vi "TeleopAuto.vi"(11 "Counts":dbl) -> ()   [LabVIEW 2018]
uses:
  <vilib>/Rock Robotics/WPI/Solenoid/WPI_SolenoidValue.ctl
  <vilib>/Rock Robotics/WPI/ThirdParty/Phoenix-LabVIEW/Motor Controller/Controls/CTRE_Phoenix_MotorControl_ControlMode.ctl
  <vilib>/Rock Robotics/WPI/Utilities/WPI_GetSetVariantRefNum.vi
  <vilib>/Rock Robotics/Network Tables/NT Write Boolean Array.vi
  <vilib>/Rock Robotics/Network Tables/NT Write Numeric Array.vi
  <vilib>/Rock Robotics/WPI/Solenoid/WPI_SolenoidSetEnum.vi
  <vilib>/Rock Robotics/Network Tables/NT Write Boolean.vi
  <vilib>/Rock Robotics/WPI/ThirdParty/Phoenix-LabVIEW/Motor Controller/Get/CTRE_Phoenix_MotorController_GetQuadratureData.vi
  <vilib>/Rock Robotics/Network Tables/NT Write Number.vi
  <vilib>/Rock Robotics/Network Tables/NT Read Number.vi
panel:
  out "Angle Ref":dbl
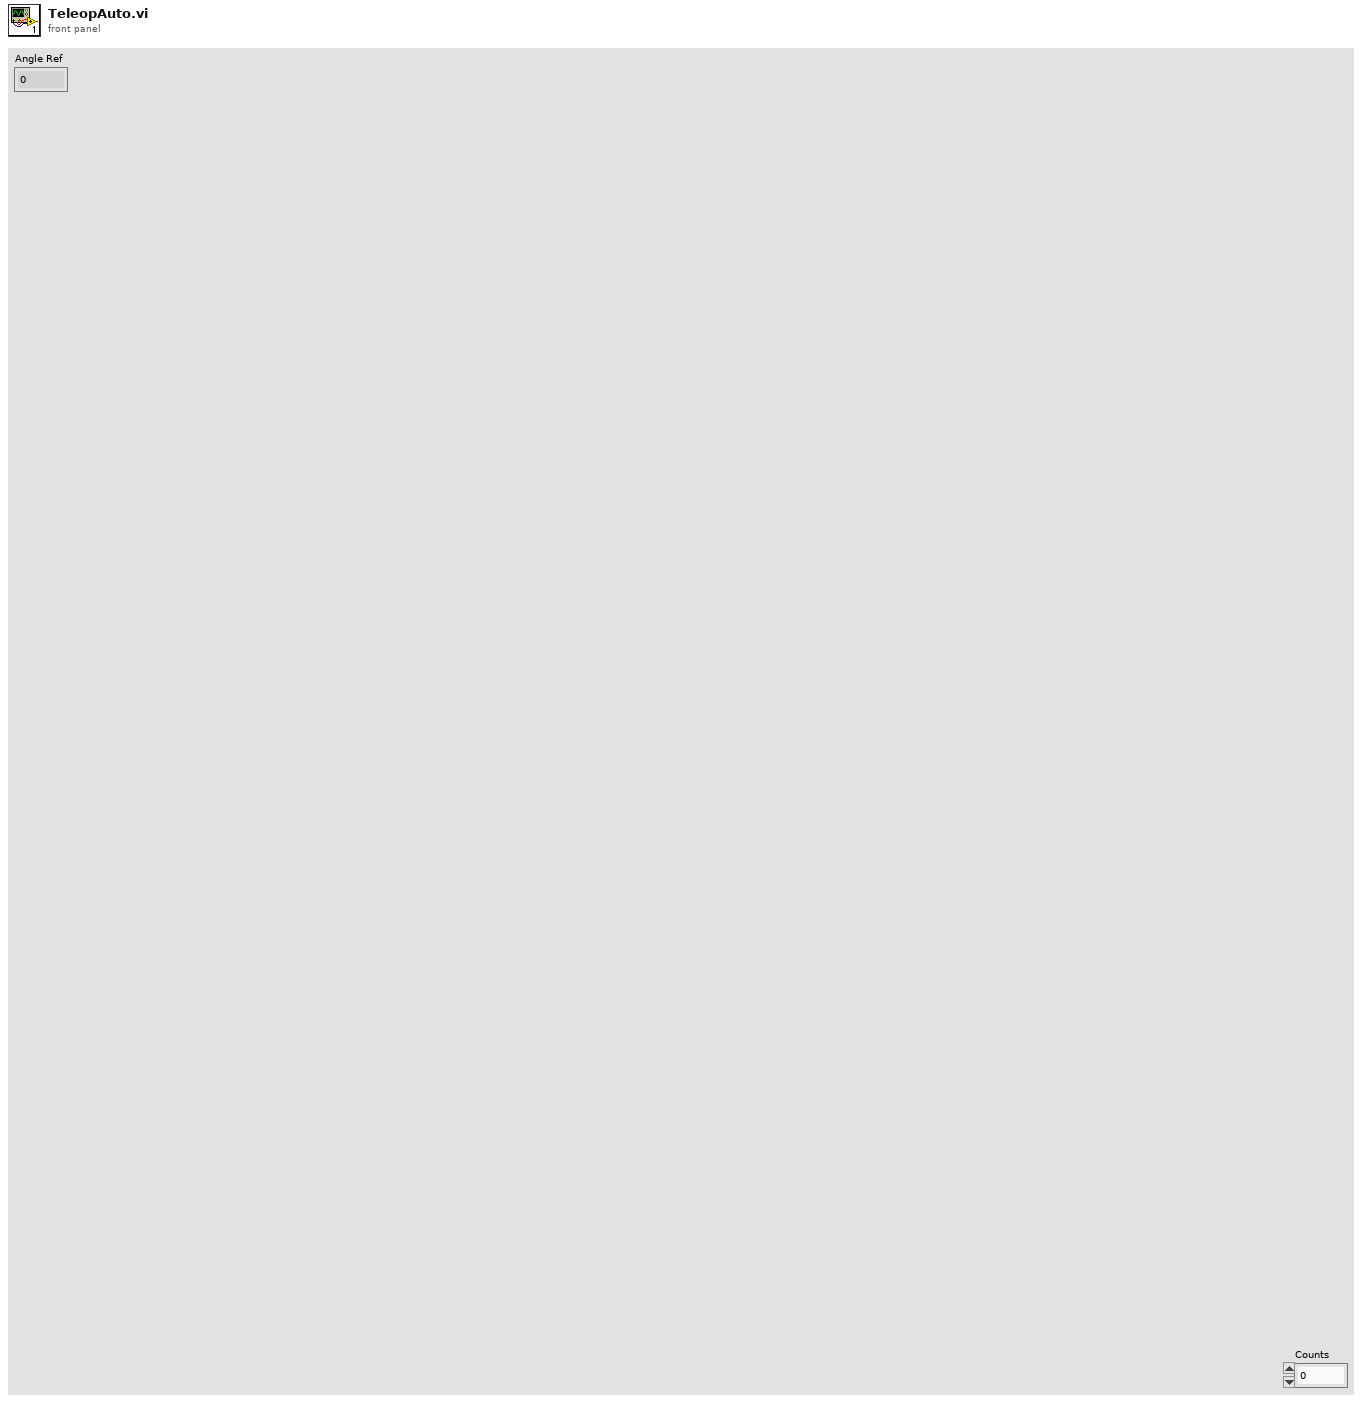
[diagram p1: front panel]
types:
  T1 = typedef "CTRE_Phoenix_MotorControl_ControlMode.ctl" = u16
  T2 = typedef "WPI_SolenoidValue.ctl" = enum16{"Off", "On", "Forward", "Reverse"}
  T3 = typedef "WPI_JoystickDevRef.ctl" = cluster{"Device":T4}
  T4 = typedef "WPI_JoystickDeviceEnum.ctl" = enum16{"USB 0", "USB 1", "USB 2", "USB 3", "USB 4", "USB 5"}
  T5 = cluster{"Buttons[0]":bool, "Buttons[1]":bool, "Buttons[2]":bool, "Buttons[3]":bool, "Buttons[4]":bool, "Buttons[5]":bool, "Buttons[6]":bool, "Buttons[7]":bool, "Buttons[8]":bool, "Buttons[9]":bool, "Buttons[10]":bool, "Buttons[11]":bool, "Buttons[12]":bool, "Buttons[13]":bool}
  T6 = cluster{"Axes[0]":dbl, "Axes[1]":dbl, "Axes[2]":dbl, "Axes[3]":dbl, "Axes[4]":dbl, "Axes[5]":dbl, "Axes[6]":dbl, "Axes[7]":dbl, "Axes[8]":dbl}
  T7 = typedef "WPI_SolenoidDevRef.ctl" = cluster{"DevStatus":errorcluster, "Pneumatics Control Module":u8, "Forward Solenoid Channel":T8, "Reverse Solenoid Channel":T8}
  T8 = typedef "WPI_SolenoidChannel.ctl" = enum8{"Solenoid 0", "Solenoid 1", "Solenoid 2", "Solenoid 3", "Solenoid 4", "Solenoid 5", "Solenoid 6", "Solenoid 7", "Invalid"}
  T9 = cluster{"Yaw":dbl, "Roll":dbl, "Pitch":dbl, "Heading":dbl, "Fused Heading":dbl}
  T10 = typedef "WPI_MotorControlDeviceRef.ctl" = cluster{"DeviceStatus":errorcluster, "Type":T11, "PWM":cluster{"PWM Channel":T12, "DeadBand":T13}, "CAN":cluster{"Device Number":u8, "SetOutput VI Ref":variant, "GetOutput VI Ref":variant, "Enable VI Ref":variant, "Disable VI Ref":variant, "Data":variant}, "Invert":bool, "DIO PWM":cluster{"PWM \"Enable\" Channel":T12, "DIOChannel":T14, "PWM Rate":dbl}}
  T11 = typedef "WPI_MotorControlType.ctl" = enum16{"PWM", "CAN", "DIO PWM"}
  T12 = typedef "FPGA_DIOPWMChannel.ctl" = enum8{"PWM 0", "PWM 1", "PWM 2", "PWM 3", "PWM 4", "PWM 5", "PWM 6", "PWM 7", "PWM 8", "PWM 9", "PWM MXP 0", "PWM MXP 1", "PWM MXP 2", "PWM MXP 3", "PWM MXP 4", "PWM MXP 5", "PWM MXP 6", "PWM MXP 7", "PWM MXP 8", "PWM MXP 9", "Invalid"}
  T13 = typedef "WPI_PWMDeadband.ctl" = cluster{"Name":string, "maxPositivePwm":i32, "minPositivePwm":i32, "centerPwm":i32, "maxNegativePwm":i32, "minNegativePwm":i32, "angularRange":u16}
  T14 = typedef "FPGA_DIOChannel.ctl" = enum8{"DIO 0", "DIO 1", "DIO 2", "DIO 3", "DIO 4", "DIO 5", "DIO 6", "DIO 7", "DIO 8", "DIO 9", "DIO MXP 0", "DIO MXP 1", "DIO MXP 2", "DIO MXP 3", "DIO MXP 4", "DIO MXP 5", "DIO MXP 6", "DIO MXP 7", "DIO MXP 8", "DIO MXP 9", "DIO MXP 10", "DIO MXP 11", "DIO MXP 12", "DIO MXP 13", "DIO MXP 14", "DIO MXP 15", "SPI Port CS1", "SPI Port CS2", "SPI Port CS3", "SPI Port MISO", "SPI Port MOSI", "Invalid"}
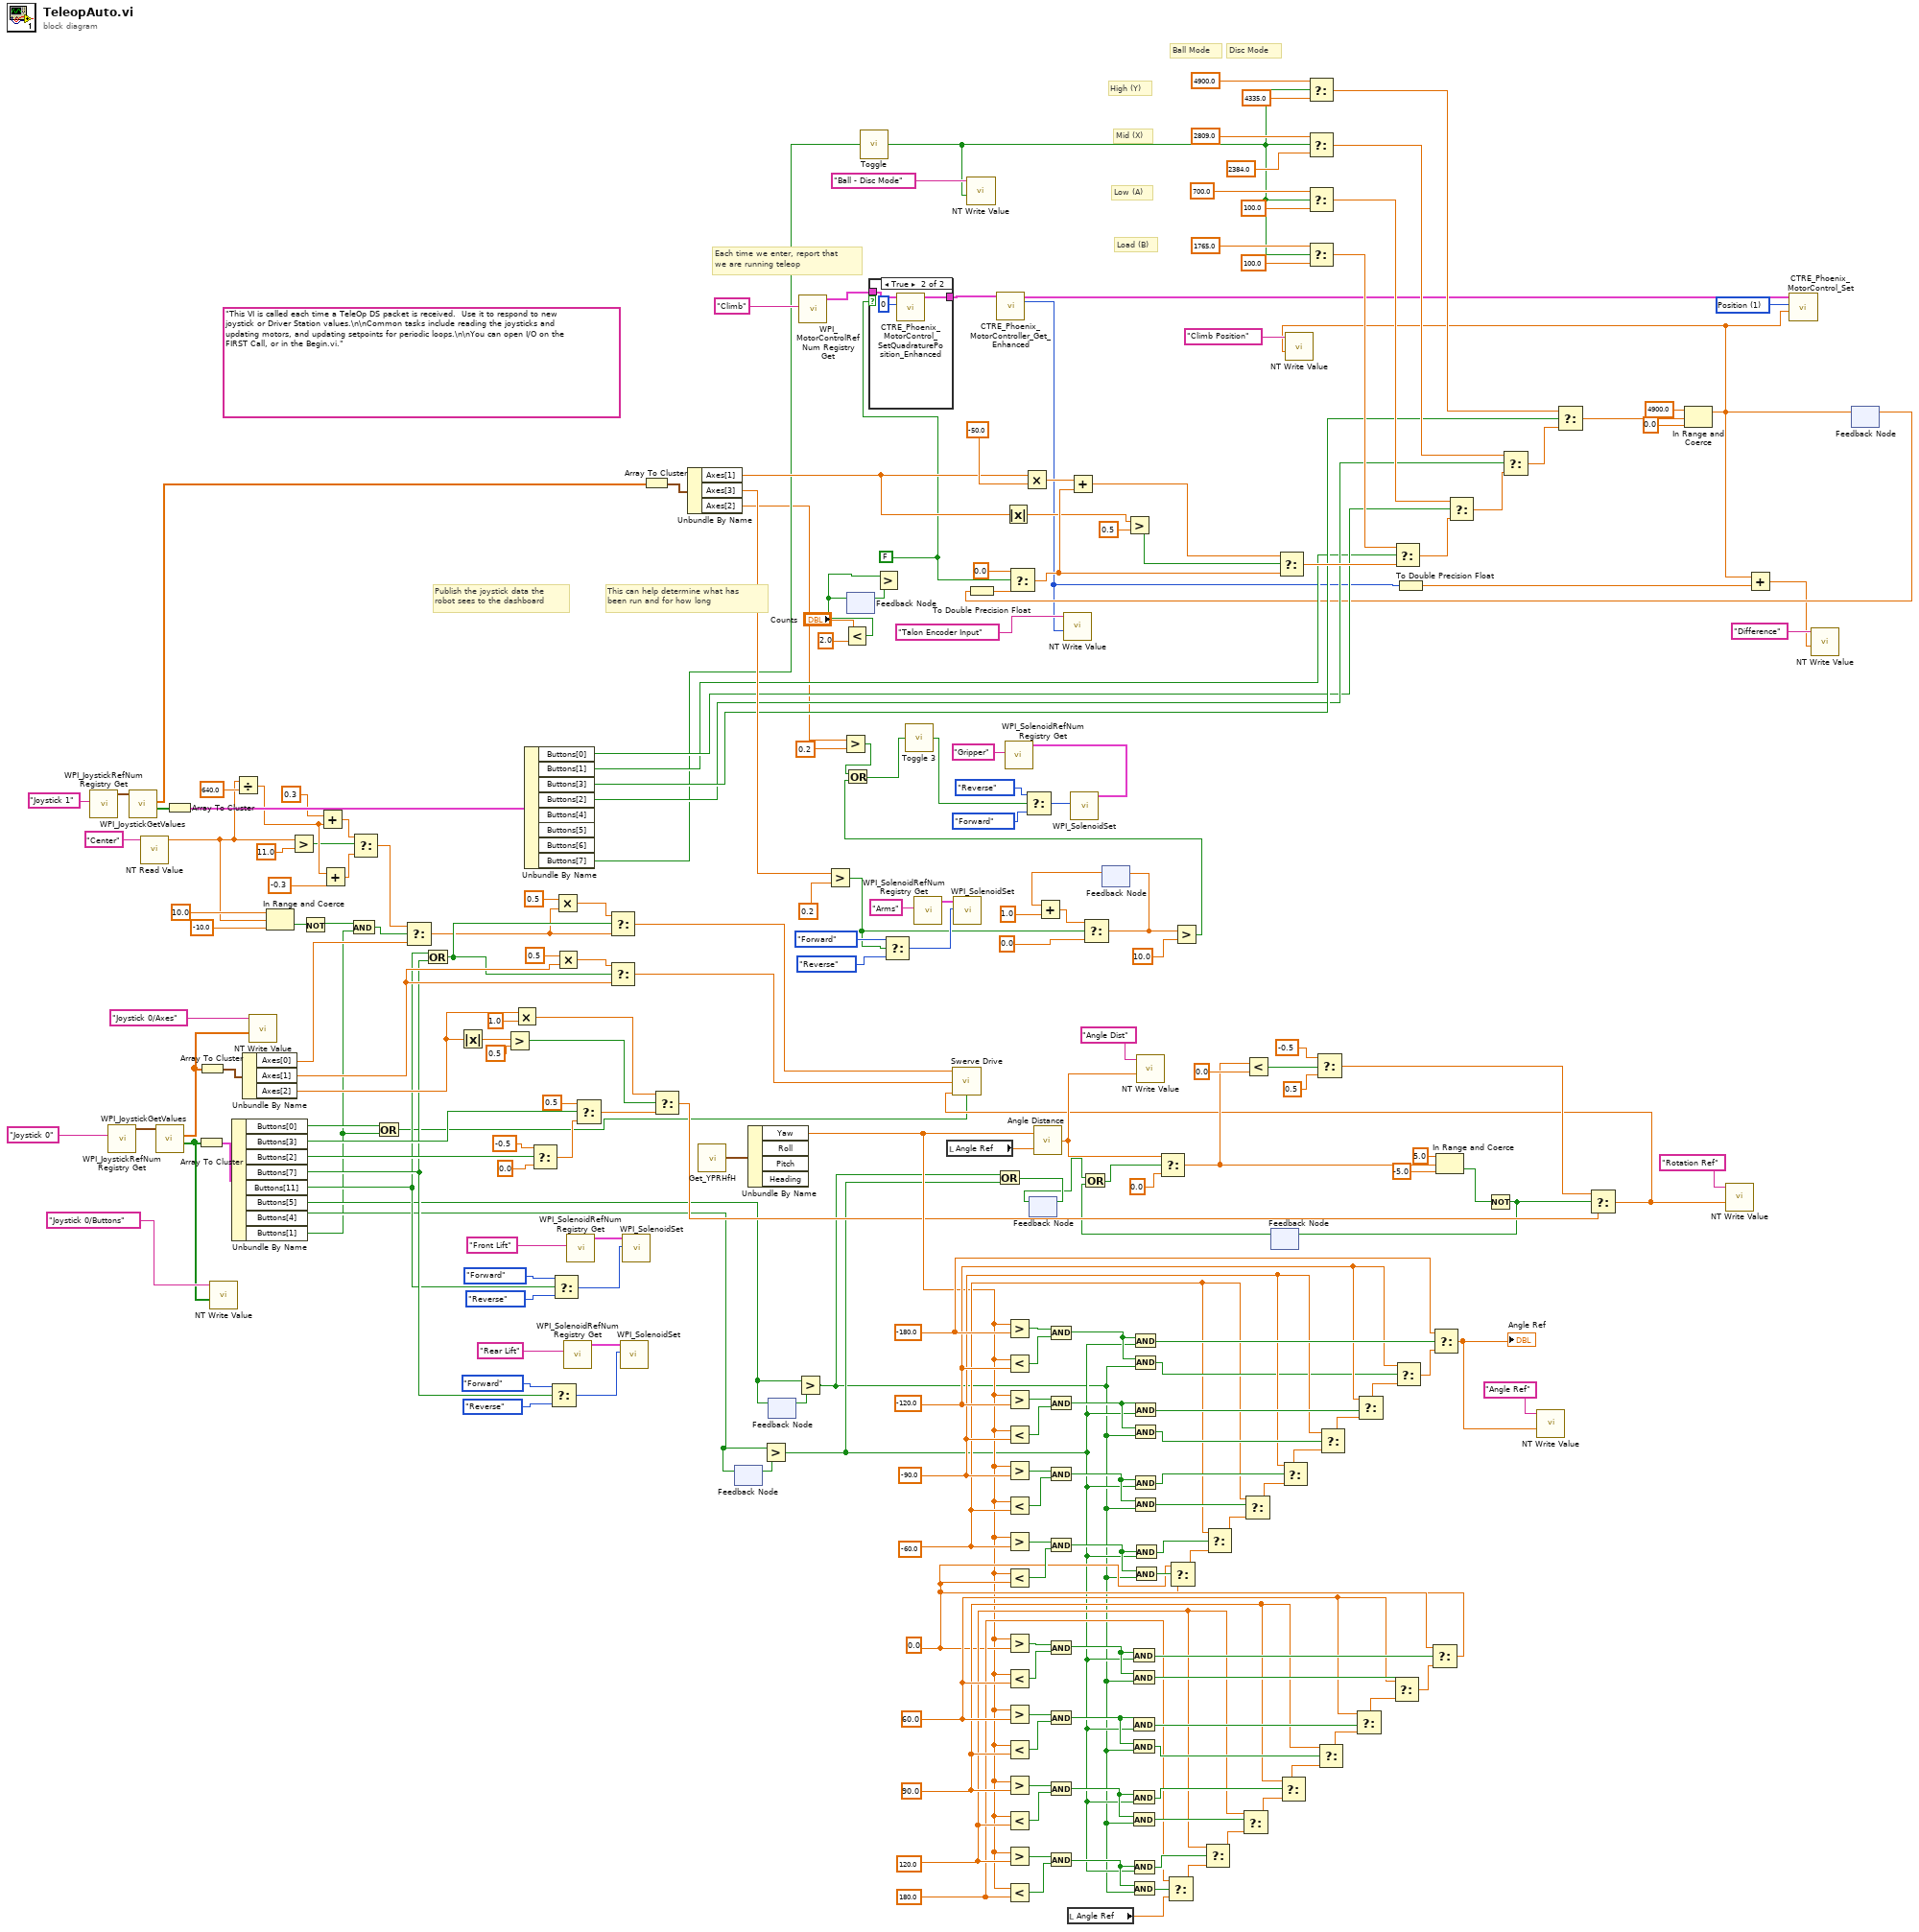
[diagram p0: block diagram]
diagram:
  w35 = FALSE
  w65 = -180.0
  w64 = -120.0
  w63 = -90.0
  w59 = -60.0
  w92 = 180.0
  w93 = 120.0
  w94 = 90.0
  w95 = 60.0
  w62 = 0.0
  w209 = T1 1 items=["PercentOutput"=0, "Position"=1, "Velocity"=2, "Current"=3, "Follower"=5, "MotionProfile"=6, "MotionMagic"=7, "MotionProfileArc"=10, "Disabled"=15] ("Control Mode")
  (unwired) "This VI is called each time a TeleOp DS packet is received.  Use it to respond to new joystick or Driver Station values.\n\nCommon tasks include reading the joysticks and updating motors, and updating setpoints for periodic loops.\n\nYou can open I/O on the FIRST Call, or in the Begin.vi."
  # "High (Y)"
  # "Mid (X)"
  # "Low (A)"
  # "Load (B)"
  # "Disc Mode"
  # "Ball Mode"
  # "Publish the joystick data the\nrobot sees to the dashboard"
  # "Each time we enter, report that\nwe are running teleop"
  # "This can help determine what has\nbeen run and for how long"
  n1 = call <vilib>:"WPI_JoystickRefNum Registry Get.vi"("refnum name"="Joystick 1") -> ("JoystickDevRef"=w216:T3)  [unwired: 1 in, 9 out]
  n2 = call <vilib>:"WPI_JoystickRefNum Registry Get.vi"("refnum name"="Joystick 0") -> ("JoystickDevRef"=w242:T3)  [unwired: 1 in, 9 out]
  n3 = call <vilib>:"WPI_JoystickGetValues.vi"("JoystickDevRef"=w216) -> ("Buttons"=w214:bool[], "Axes"=w210:dbl[])  [unwired: 6 in, 3 out]
  n4 = call-poly <vilib>:"NT Read Value.vi"("Name"="Center" ("refnum name")) -> ("Numeric"=w6:dbl)  [unwired: 9 in, 1 out]
  n5 = call <vilib>:"WPI_JoystickGetValues.vi"("JoystickDevRef"=w242) -> ("Buttons"=w237:bool[], "Axes"=w239:dbl[])  [unwired: 6 in, 3 out]
  n6 = Array To Cluster(array=w214) -> (cluster=w213:T5)
  n7 = Array To Cluster(array=w237) -> (cluster=w236:T5)
  n8 = Array To Cluster(array=w239) -> (cluster=w238:T6)
  n9 = call-poly <vilib>:"NT Write Value.vi"("Boolean Array"=w237, "Name"="Joystick 0/Buttons") -> ()  [unwired: 9 in, 1 out]
  n10 = Unbundle By Name(w236) -> ("Buttons[0]"=w20:bool, "Buttons[3]"=w134:bool, "Buttons[2]"=w135:bool, "Buttons[7]"=w52:bool, "Buttons[11]"=w51:bool, "Buttons[5]"=w34:bool, "Buttons[4]"=w32:bool, "Buttons[1]"=w16:bool)
  n11 = Divide(x=w6, y=640.0) -> (x/y=w5:dbl)
  n12 = Unbundle By Name(w238) -> ("Axes[0]"=w24:dbl, "Axes[1]"=w54:dbl, "Axes[2]"=w141:dbl)
  n13 = call-poly <vilib>:"NT Write Value.vi"("Numeric Array"=w239, "Name"="Joystick 0/Axes") -> ()  [unwired: 9 in, 1 out]
  n14 = In Range and Coerce(upper limit=10.0, x=w6, lower limit=-10.0) -> (In Range?=w14:bool)  [unwired: 1 out]
  n15 = Greater?(x=w6, y=11.0) -> (0:w4:bool)
  n16 = Not(x=w14) -> (.not. x?=w15:bool)
  n17 = Add(x=0.3 ("t"), y=w5) -> (x+y=w10:dbl)
  n18 = Add(x=w5, y=-0.3 ("f")) -> (x+y=w11:dbl)
  n19 = And(x=w15, y=w16) -> (x .and. y?=w13:bool)
  n20 = Select(t=w10, s=w4, f=w11) -> (s? t:f=w22:dbl)
  n21 = Or(x=w20, y=w16) -> (x .or. y?=w19:bool)
  n22 = Select(t=w22, s=w13, f=w24) -> (s? t:f=w23:dbl)
  n23 = Or(x=w51, y=w52) -> (x .or. y?=w50:bool)
  n24 = Absolute Value(x=w141) -> (abs(x)=w144:dbl)
  n25 = Greater?(x=w144, y=0.5) -> (0:w133:bool)
  n26 = Multiply(x=w141, y=1.0) -> (x*y=w142:dbl)
  n27 = Unbundle By Name(w213) -> ("Buttons[0]"=w175:bool, "Buttons[1]"=w174:bool, "Buttons[3]"=w177:bool, "Buttons[2]"=w176:bool, "Buttons[7]"=w172:bool)  [unwired: 3 out]
  n28 = Select(t=-0.5, s=w135, f=0.0) -> (s? t:f=w139:dbl)
  n29 = Select(t=WPI_SolenoidValue."Forward" ("Value"), s=w52, f=WPI_SolenoidValue."Reverse") -> (s? t:f=w219:T2)
  n30 = Select(t=WPI_SolenoidValue."Forward" ("Value"), s=w51, f=WPI_SolenoidValue."Reverse") -> (s? t:f=w218:T2)
  n31 = Multiply(x=0.5, y=w23) -> (x*y=w53:dbl)
  n32 = Multiply(x=0.5, y=w54) -> (x*y=w55:dbl)
  n33 = call <vilib>:"WPI_SolenoidRefNum Registry Get.vi"("refnum name"="Rear Lift") -> ("SolenoidDevRef"=w229:T7)  [unwired: 9 in, 1 out]
  n34 = call <vilib>:"WPI_SolenoidRefNum Registry Get.vi"("refnum name"="Front Lift") -> ("SolenoidDevRef"=w230:T7)  [unwired: 9 in, 1 out]
  n35 = Select(t=0.5, s=w134, f=w139) -> (s? t:f=w132:dbl)
  n36 = Select(t=w53, s=w50, f=w23) -> (s? t:f=w48:dbl)
  n37 = Select(t=w55, s=w50, f=w54) -> (s? t:f=w49:dbl)
  n38 = call-poly <vilib>:"WPI_SolenoidSet.vi"("Value"=w219, "SolenoidDevRef"=w229) -> ()  [unwired: 8 in, 2 out]
  n39 = call-poly <vilib>:"WPI_SolenoidSet.vi"("Value"=w218, "SolenoidDevRef"=w230) -> ()  [unwired: 8 in, 2 out]
  n40 = Array To Cluster(array=w210) -> (cluster=w211:T6)
  n41 = Select(t=w142, s=w133, f=w132) -> (s? t:f=w43:dbl)
  n42 = Unbundle By Name(w211) -> ("Axes[1]"=w197:dbl, "Axes[3]"=w204:dbl, "Axes[2]"=w170:dbl)
  n43 = call <vilib>:"Get_YPRHfH.vi"() -> ("YRPHfH"=w131:T9)  [unwired: 11 in]
  n44 = feedback #1() -> (w45:bool)  [unwired: 1 in]
  n45 = feedback-in #1(w32) -> ()
  n46 = Unbundle By Name(w131) -> ("Yaw"=w58:dbl)  [unwired: 3 out]
  n47 = Greater?(x=w32, y=w45) -> (0:w26:bool)
  n48 = feedback #2() -> (w46:bool)  [unwired: 1 in]
  n49 = feedback-in #2(w34) -> ()
  n50 = Greater?(x=w34, y=w46) -> (0:w25:bool)
  n51 = call <vilib>:"WPI_MotorControlRefNum Registry Get.vi"("refnum name"="Climb") -> ("MotorControlDevRef"=w155:T10)  [unwired: 9 in, 1 out]
  n52 = Greater?(x=w204, y=0.2) -> (0:w167:bool)
  n53 = Greater?(x=w170, y=0.2) -> (0:w160:bool)
  n54 = Less?(x="Counts", y=2.0) -> (x < y?=w2:bool)
  n55 = feedback #3() -> (w153:bool)  [unwired: 1 in]
  n56 = feedback-in #3(w2) -> ()
  n57 = call "Toggle.vi"("Input"=w172) -> ("Output"=w157:bool)
  n58 = case shown="True" w35 {
    tunnel: w155 -> [w244 w247]
    tunnel: [w244 w246] -> w154
    frame False {
    }
    frame True {
      n59 = call <vilib>:"CTRE_Phoenix_MotorControl_SetQuadraturePosition_Enhanced.vi"("New Position"=0, "PhoenixMotorControlDevRef"=w247) -> ("PhoenixMotorControlDevRef"=w246:T10)  [unwired: 8 in, 1 out]
    }
  }
  n60 = Greater?(x=w2, y=w153) -> ()  [unwired: 1 out]
  n61 = Select(t=WPI_SolenoidValue."Forward" ("Value"), s=w167, f=WPI_SolenoidValue."Reverse") -> (s? t:f=w232:T2)
  n62 = call <vilib>:"WPI_SolenoidRefNum Registry Get.vi"("refnum name"="Arms") -> ("SolenoidDevRef"=w234:T7)  [unwired: 9 in, 1 out]
  n63 = local read "Angle Ref"() -> (w47:dbl)
  n64 = call-poly <vilib>:"WPI_SolenoidSet.vi"("Value"=w232, "SolenoidDevRef"=w234) -> ()  [unwired: 8 in, 2 out]
  n65 = call-poly <vilib>:"NT Write Value.vi"("Boolean"=w157, "Name"="Ball - Disc Mode") -> ()  [unwired: 9 in, 1 out]
  n66 = Or(x=w25, y=w26) -> (x .or. y?=w28:bool)
  n67 = call-poly <vilib>:"CTRE_Phoenix_MotorController_Get_Enhanced.vi"("PhoenixMotorControlDevRef"=w154) -> ("PhoenixMotorControlDevRef"=w158:T10, "Quadrature Position"=w148:i32)  [unwired: 11 in, 2 out]
  n68 = Absolute Value(x=w197) -> (abs(x)=w196:dbl)
  n69 = call <vilib>:"WPI_SolenoidRefNum Registry Get.vi"("refnum name"="Gripper") -> ("SolenoidDevRef"=w231:T7)  [unwired: 9 in, 1 out]
  n70 = Greater?(x=w58, y=w65) -> (0:w91:bool)
  n71 = Less?(x=w58, y=w64) -> (x < y?=w90:bool)
  n72 = Greater?(x=w58, y=w64) -> (0:w86:bool)
  n73 = Less?(x=w58, y=w63) -> (x < y?=w85:bool)
  n74 = Greater?(x=w58, y=w63) -> (0:w84:bool)
  n75 = Less?(x=w58, y=w59) -> (x < y?=w83:bool)
  n76 = Greater?(x=w58, y=w59) -> (0:w82:bool)
  n77 = Less?(x=w58, y=w62) -> (x < y?=w81:bool)
  n78 = Greater?(x=w58, y=w62) -> (0:w122:bool)
  n79 = Less?(x=w58, y=w95) -> (x < y?=w121:bool)
  n80 = Greater?(x=w58, y=w95) -> (0:w116:bool)
  n81 = Less?(x=w58, y=w94) -> (x < y?=w115:bool)
  n82 = Greater?(x=w58, y=w94) -> (0:w114:bool)
  n83 = Less?(x=w58, y=w93) -> (x < y?=w113:bool)
  n84 = Greater?(x=w58, y=w93) -> (0:w112:bool)
  n85 = Less?(x=w58, y=w92) -> (x < y?=w111:bool)
  n86 = Multiply(x=w197, y=-50.0) -> (x*y=w202:dbl)
  n87 = feedback #4() -> (w27:bool)  [unwired: 1 in]
  n88 = feedback-in #4(w28) -> ()
  n89 = call "Angle Distance.vi"("target angle"=w47, "current angle"=w58) -> ("distance"=w38:dbl)
  n90 = And(x=w91, y=w90) -> (x .and. y?=w89:bool)
  n91 = And(x=w86, y=w85) -> (x .and. y?=w80:bool)
  n92 = And(x=w84, y=w83) -> (x .and. y?=w79:bool)
  n93 = And(x=w82, y=w81) -> (x .and. y?=w78:bool)
  n94 = And(x=w122, y=w121) -> (x .and. y?=w120:bool)
  n95 = And(x=w116, y=w115) -> (x .and. y?=w110:bool)
  n96 = And(x=w114, y=w113) -> (x .and. y?=w109:bool)
  n97 = And(x=w112, y=w111) -> (x .and. y?=w108:bool)
  n98 = call-poly <vilib>:"NT Write Value.vi"("Numeric"=w148, "Name"="Talon Encoder Input") -> ()  [unwired: 9 in, 1 out]
  n99 = local read "Angle Ref"() -> (w33:dbl)
  n100 = feedback #5() -> (w163:dbl)  [unwired: 1 in]
  n101 = Add(x=w163, y=1.0) -> (x+y=w165:dbl)
  n102 = Select(t=w165, s=w167, f=0.0) -> (s? t:f=w162:dbl)
  n103 = feedback-in #5(w162) -> ()
  n104 = Greater?(x=w196, y=0.5) -> (0:w195:bool)
  n105 = And(x=w120, y=w26) -> (x .and. y?=w119:bool)
  n106 = And(x=w120, y=w25) -> (x .and. y?=w118:bool)
  n107 = And(x=w110, y=w26) -> (x .and. y?=w101:bool)
  n108 = And(x=w110, y=w25) -> (x .and. y?=w100:bool)
  n109 = And(x=w109, y=w26) -> (x .and. y?=w99:bool)
  n110 = And(x=w109, y=w25) -> (x .and. y?=w98:bool)
  n111 = And(x=w108, y=w26) -> (x .and. y?=w97:bool)
  n112 = And(x=w108, y=w25) -> (x .and. y?=w96:bool)
  n113 = And(x=w89, y=w26) -> (x .and. y?=w88:bool)
  n114 = And(x=w89, y=w25) -> (x .and. y?=w60:bool)
  n115 = And(x=w80, y=w26) -> (x .and. y?=w71:bool)
  n116 = And(x=w80, y=w25) -> (x .and. y?=w70:bool)
  n117 = And(x=w79, y=w26) -> (x .and. y?=w69:bool)
  n118 = And(x=w79, y=w25) -> (x .and. y?=w68:bool)
  n119 = And(x=w78, y=w26) -> (x .and. y?=w67:bool)
  n120 = And(x=w78, y=w25) -> (x .and. y?=w66:bool)
  n121 = call-poly <vilib>:"NT Write Value.vi"("Numeric"=w38, "Name"="Angle Dist") -> ()  [unwired: 9 in, 1 out]
  n122 = Select(t=w92, s=w96, f=w33) -> (s? t:f=w102:dbl)
  n123 = Greater?(x=w162, y=10.0) -> (0:w159:bool)
  n124 = Or(x=w160, y=w159) -> (x .or. y?=w1:bool)
  n125 = call "Toggle 3.vi"("Input"=w1) -> ("Output"=w168:bool)
  n126 = Select(t=WPI_SolenoidValue."Reverse" ("Value"), s=w168, f=WPI_SolenoidValue."Forward") -> (s? t:f=w217:T2)
  n127 = call-poly <vilib>:"WPI_SolenoidSet.vi"("Value"=w217, "SolenoidDevRef"=w231) -> ()  [unwired: 8 in, 2 out]
  n128 = Select(t=w93, s=w97, f=w102) -> (s? t:f=w103:dbl)
  n129 = Select(t=w93, s=w98, f=w103) -> (s? t:f=w104:dbl)
  n130 = feedback #6() -> (w30:bool)  [unwired: 1 in]
  n131 = Or(x=w27, y=w30) -> (x .or. y?=w29:bool)
  n132 = Select(t=w38, s=w29, f=0.0) -> (s? t:f=w126:dbl)
  n133 = Less?(x=w126, y=0.0) -> (x < y?=w125:bool)
  n134 = Select(t=w94, s=w99, f=w104) -> (s? t:f=w105:dbl)
  n135 = Select(t=4900.0, s=w157, f=4335.0) -> (s? t:f=w188:dbl)
  n136 = Select(t=2809.0, s=w157, f=2384.0) -> (s? t:f=w189:dbl)
  n137 = Select(t=700.0, s=w157, f=100.0) -> (s? t:f=w190:dbl)
  n138 = Select(t=1765.0, s=w157, f=100.0) -> (s? t:f=w191:dbl)
  n139 = Select(t=-0.5, s=w125, f=0.5) -> (s? t:f=w42:dbl)
  n140 = Select(t=w94, s=w100, f=w105) -> (s? t:f=w106:dbl)
  n141 = Select(t=w95, s=w101, f=w106) -> (s? t:f=w107:dbl)
  n142 = Select(t=w95, s=w118, f=w107) -> (s? t:f=w117:dbl)
  n143 = To Double Precision Float(number=w148) -> (double precision float=w147:dbl)
  n144 = Select(t=w62, s=w119, f=w117) -> (s? t:f=w61:dbl)
  n145 = Select(t=w62, s=w66, f=w61) -> (s? t:f=w72:dbl)
  n146 = Select(t=w59, s=w67, f=w72) -> (s? t:f=w73:dbl)
  n147 = Select(t=w59, s=w68, f=w73) -> (s? t:f=w74:dbl)
  n148 = Select(t=w63, s=w69, f=w74) -> (s? t:f=w75:dbl)
  n149 = Select(t=w63, s=w70, f=w75) -> (s? t:f=w76:dbl)
  n150 = Select(t=w64, s=w71, f=w76) -> (s? t:f=w77:dbl)
  n151 = Select(t=w64, s=w60, f=w77) -> (s? t:f=w87:dbl)
  n152 = Select(t=w65, s=w88, f=w87) -> (s? t:f=w40:dbl)
  "Angle Ref" <- w40
  n153 = In Range and Coerce(upper limit=5.0, x=w126, lower limit=-5.0) -> (In Range?=w44:bool)  [unwired: 1 out]
  n154 = Not(x=w44) -> (.not. x?=w31:bool)
  n155 = feedback-in #6(w31) -> ()
  n156 = call-poly <vilib>:"NT Write Value.vi"("Numeric"=w40, "Name"="Angle Ref") -> ()  [unwired: 9 in, 1 out]
  n157 = Select(t=w42, s=w31, f=w43) -> (s? t:f=w36:dbl)
  n158 = call "Swerve Drive.vi"("X"=w48, "Y"=w49, "Z"=w36, "Robot-Centric"=w19) -> ()  [unwired: 12 in]
  n159 = call-poly <vilib>:"NT Write Value.vi"("Numeric"=w36, "Name"="Rotation Ref") -> ()  [unwired: 9 in, 1 out]
  n160 = feedback #7() -> (w150:dbl)  [unwired: 1 in]
  n161 = To Double Precision Float(number=w150) -> (double precision float=w151:dbl)
  n162 = Select(t=0.0, s=w35, f=w151) -> (s? t:f=w198:dbl)
  n163 = Add(x=w202, y=w198) -> (x+y=w199:dbl)
  n164 = Select(t=w199, s=w195, f=w198) -> (s? t:f=w187:dbl)
  n165 = Select(t=w191, s=w174, f=w187) -> (s? t:f=w194:dbl)
  n166 = Select(t=w190, s=w175, f=w194) -> (s? t:f=w193:dbl)
  n167 = Select(t=w189, s=w176, f=w193) -> (s? t:f=w192:dbl)
  n168 = Select(t=w188, s=w177, f=w192) -> (s? t:f=w186:dbl)
  n169 = In Range and Coerce(upper limit=4900.0, x=w186, lower limit=0.0) -> (coerced(x)=w149:dbl)  [unwired: 1 out]
  n170 = call-poly <vilib>:"NT Write Value.vi"("Numeric"=w149, "Name"="Climb Position") -> ()  [unwired: 9 in, 1 out]
  n171 = Add(x=w149, y=w147) -> (x+y=w145:dbl)
  n172 = call <vilib>:"CTRE_Phoenix_MotorControl_Set.vi"("Output"=w149, "Control Mode"=w209, "PhoenixMotorControlDevRef"=w158) -> ()  [unwired: 7 in, 2 out]
  n173 = call-poly <vilib>:"NT Write Value.vi"("Numeric"=w145, "Name"="Difference") -> ()  [unwired: 9 in, 1 out]
  n174 = feedback-in #7(w149) -> ()
